vi "Quaternion to Rotation Matrix.vi"(8 "error in (no error)":errorcluster, 11 "Quaternion":T2) -> (0 "error out":errorcluster, 3 "Rotation Matrix":T1)   [LabVIEW 2020, in "g_ar_toolkit.ar.lvlib"]
uses:
  g_ar_toolkit.ar.lvlib
  Quaternion.ctl
  <vilib>/Analysis/Matrix/Datatypes/RealMatrix.ctl
  <vilib>/Analysis/Matrix/Numeric/Conversions/Array To Matrix - RA2.vi
  <vilib>/Analysis/Matrix/NI_Matrix.lvlib
  g_ar_toolkit.common/g_ar_toolkit.common.lvlib
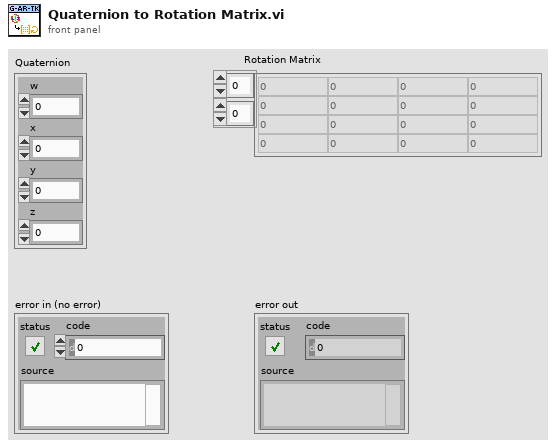
[diagram p1: front panel]
types:
  T1 = typedef "NI_Matrix.lvlib/RealMatrix.ctl" = dbl[][]
  T2 = typedef "g_ar_toolkit.ar.lvlib/Quaternion.ctl" = cluster{"w":dbl, "x":dbl, "y":dbl, "z":dbl}
  T3 = cluster{"m 0,0":dbl, "m 0,1":dbl, "m 0,2":dbl, "m 1,0":dbl, "m 1,1":dbl, "m 1,2":dbl, "m 2,0":dbl, "m 2,1":dbl, "m 2,2":dbl}
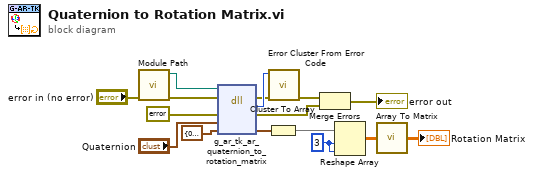
[diagram p0: block diagram]
diagram:
  w5 = 3 ("dimension size")
  n1 = call "Module Path.vi"("error in (no error)"="error in (no error)") -> ("error out"=w2:errorcluster, "Path"=w1:path)  [unwired: 9 in]
  n2 = dll-call lib="?" fn="g_ar_tk_ar_quaternion_to_rotation_matrix" ("g_ar_toolkit.*.*:g_ar_tk_image_copy")(path in=w1, error in=w2, "error_cluster"=errorcluster {"status"=FALSE, "code"=0, "source"=""} ("error constant"), "quaternion"="Quaternion", "rmat"=T3 {"m 0,0"=0.0, "m 0,1"=0.0, "m 0,2"=0.0, "m 1,0"=0.0, "m 1,1"=0.0, "m 1,2"=0.0, "m 2,0"=0.0, "m 2,1"=0.0, "m 2,2"=0.0} ("Matrix")) -> (error out=w11:errorcluster, "MgErr"=w12:i32, "error_cluster"=w15:errorcluster, "rmat"=w7:T3)  [unwired: 2 in, 1 out]
  n3 = Cluster To Array(cluster=w7) -> (array=w6:dbl[])
  n4 = call <vilib>:"Error Cluster From Error Code.vi"("error in (no error)"=w11, "error code (0)"=w12) -> ("error out"=w13:errorcluster)  [unwired: 7 in]
  n5 = Merge Errors(w13, w15) -> (→"error out":errorcluster)
  n6 = Reshape Array(w6, w5, w5) -> (w4:dbl[][])
  n7 = call-poly <vilib>:"Array To Matrix.vi"("Real 2D Array"=w4) -> ("Real Matrix"=→"Rotation Matrix":T1)
